vi "channel_data_to_array.vi"(0 "Channel 1 Pressures Array":dbl[](array[numeric]), 1 "Channel 1 Pressure":dbl, 2 "Max Array Size":i32, 3 "Channel 2 Pressure":dbl, 11 "Channel 2 Pressures Array":dbl[](array[numeric])) -> (4 "Channel 1 Pressures Array Out":dbl[](array[numeric]), 12 "Channel 1 XY data":cluster{i32[], dbl[]}, 14 "Channel 2 XY data":cluster{i32[], dbl[]}, 15 "Channel 2 Pressures Array Out":dbl[](array[numeric]))   [LabVIEW 2019]
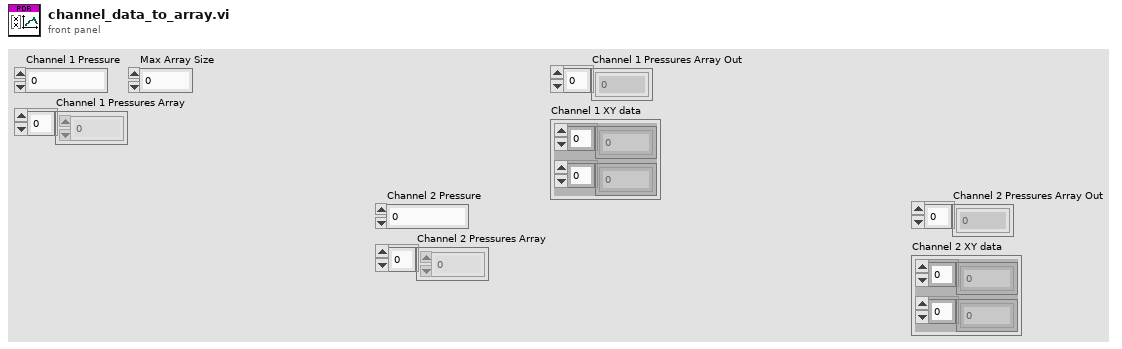
[diagram p1: front panel]
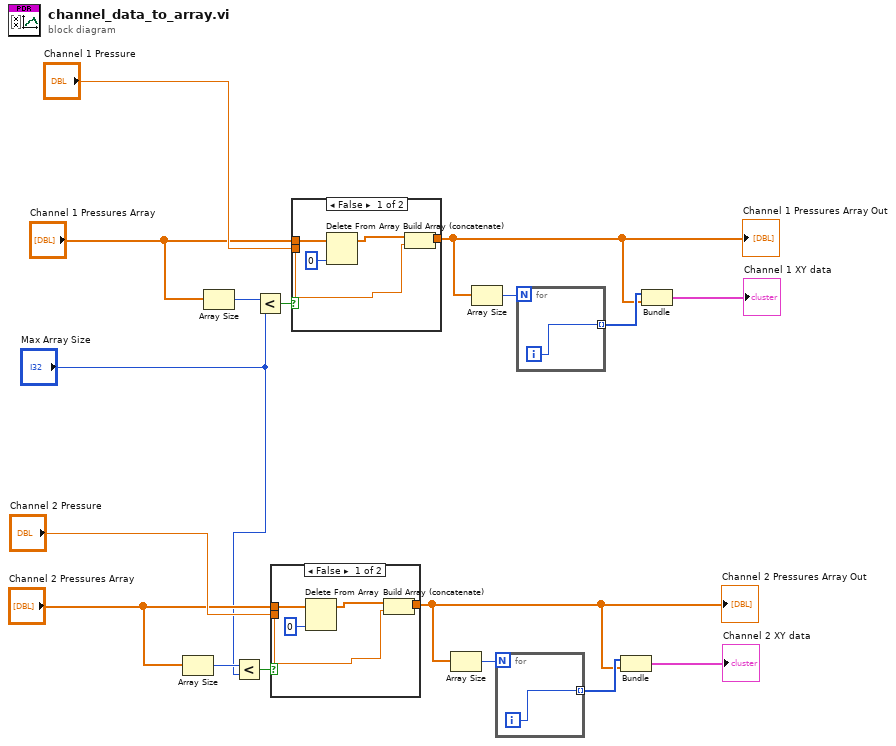
[diagram p0: block diagram]
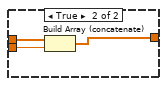
[diagram p2: hidden frame]
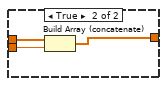
[diagram p3: hidden frame]
diagram:
  n1 = Array Size(array="Channel 2 Pressures Array") -> (size(s)=w8:i32)
  n2 = Array Size(array="Channel 1 Pressures Array") -> (size(s)=w16:i32)
  n3 = Less?(x=w8, y="Max Array Size") -> (x < y?=w9:bool)
  n4 = Less?(x=w16, y="Max Array Size") -> (x < y?=w17:bool)
  n5 = case shown="False" w9 {
    tunnel: "Channel 2 Pressures Array" -> [w22 w25]
    tunnel: "Channel 2 Pressure" -> [w19 w24]
    tunnel: [w20 w23] -> w5
    frame False {
      n6 = Delete From Array(array=w22, index=0) -> (array with subset deleted=w18:dbl[])  [unwired: 1 in, 1 out]
      n7 = Build Array (concatenate)(w18, w19) -> (w20:dbl[])
    }
    frame True {
      n8 = Build Array (concatenate)(w25, w24) -> (w23:dbl[])
    }
  }
  "Channel 2 Pressures Array Out" <- w5
  n9 = case shown="False" w17 {
    tunnel: "Channel 1 Pressures Array" -> [w30 w33]
    tunnel: "Channel 1 Pressure" -> [w27 w32]
    tunnel: [w28 w31] -> w13
    frame False {
      n10 = Delete From Array(array=w30, index=0) -> (array with subset deleted=w26:dbl[])  [unwired: 1 in, 1 out]
      n11 = Build Array (concatenate)(w26, w27) -> (w28:dbl[])
    }
    frame True {
      n12 = Build Array (concatenate)(w33, w32) -> (w31:dbl[])
    }
  }
  "Channel 1 Pressures Array Out" <- w13
  n13 = Array Size(array=w5) -> (size(s)=w7:i32)
  n14 = Array Size(array=w13) -> (size(s)=w15:i32)
  n15 = for {
    N: w7 -> [_]
    tunnel: [w34] -> w6 mode=indexing
    i -> [w34]
  }
  n16 = for {
    N: w15 -> [_]
    tunnel: [w35] -> w14 mode=indexing
    i -> [w35]
  }
  n17 = Bundle(w6, w5) -> (→"Channel 2 XY data":cluster{i32[], dbl[]})  [unwired: 1 in]
  n18 = Bundle(w14, w13) -> (→"Channel 1 XY data":cluster{i32[], dbl[]})  [unwired: 1 in]
